vi "TestSerial.vi"() -> ()   [LabVIEW 2016]
uses:
  <vilib>/Instr/_visa.llb/VISA Configure Serial Port (Instr).vi
panel:
  out "Time":u32
  out "millisecond timer value":u32
  out "return count 2":u32
  out "unsigned byte array":u8[](array[numeric])
  out "return count":u32
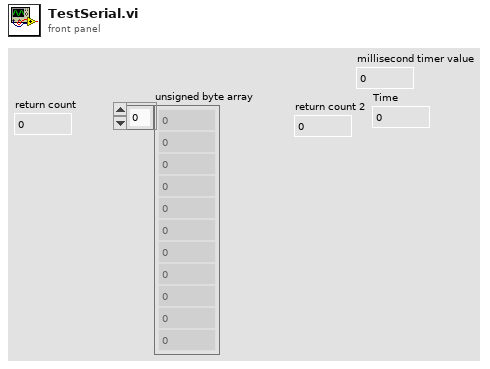
[diagram p1: front panel]
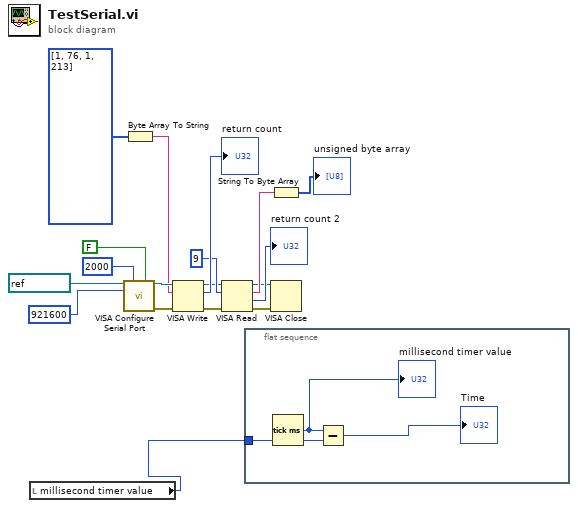
[diagram p0: block diagram]
diagram:
  n1 = local read "millisecond timer value"() -> (w1:u32)
  n2 = call-poly "VISA Configure Serial Port"("VISA resource name"=refnum<visa-resource-name> "COM6", "timeout (10sec)"=u32 2000, "Enable Termination\nChar (T)"=FALSE ("Enable Termination\nChar (T)"), "baud rate (9600)"=u32 921600) -> ("VISA resource name out"=w12:refnum<visa-resource-name>, "error out"=w13:errorcluster)  [unwired: 10 in]
  n3 = Byte Array To String(unsigned byte array=u8[] [1, 76, 1, 213]) -> (string=w11:string)
  n4 = VISA Write(VISA resource name=w12, write buffer=w11, error in (no error)=w13) -> (VISA resource name out=w7:refnum<visa-resource-name>, return count=→"return count":u32, error out=w9:errorcluster)
  n5 = VISA Read(VISA resource name=w7, byte count=u32 9, error in (no error)=w9) -> (VISA resource name out=w2:refnum<visa-resource-name>, read buffer=w6:string, return count=→"return count 2":u32, error out=w3:errorcluster)
  n6 = flat-sequence {
    tunnel: w1 -> [w20]
    frame #0 {
      n7 = Tick Count (ms)() -> (millisecond timer value=w21:u32)
      "millisecond timer value" <- w21
      n8 = Subtract(x=w21, y=w20) -> (x-y=→"Time":u32)
    }
  }
  n9 = String To Byte Array(string=w6) -> (unsigned byte array=→"unsigned byte array":u8[])
  n10 = VISA Close(VISA resource name=w2, error in (no error)=w3) -> ()  [unwired: 1 out]
